vi "Umfang.vi"(9 "Breite":dbl, 10 "Länge":dbl, 11 "error in (no error)":errorcluster) -> (1 "error out":errorcluster, 2 "Umfang":dbl)   [LabVIEW 2024]
doc: "Berechnet den Umfang eines Rechteckes"
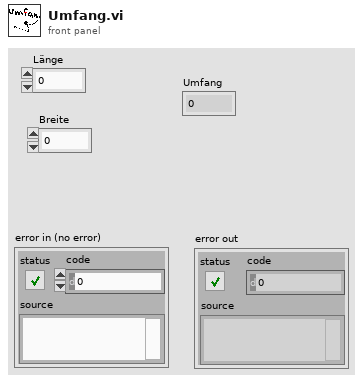
[diagram p1: front panel]
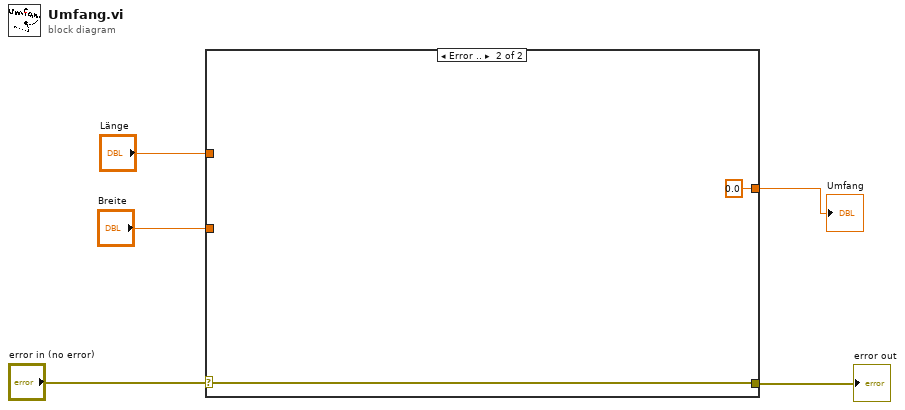
[diagram p0: block diagram]
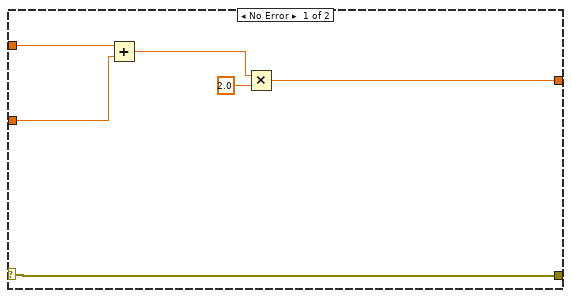
[diagram p2: hidden frame]
diagram:
  n1 = case shown="Error .." "error in (no error)" {
    selector: "error in (no error)" -> [w11 w12]
    tunnel: [w11 w12] -> w4
    tunnel: "Länge" -> [w10 _]
    tunnel: "Breite" -> [w9 _]
    tunnel: [w6 0.0] -> w1
    frame No Error {
      n2 = Add(x=w10, y=w9) -> (x+y=w8:dbl)
      n3 = Multiply(x=w8, y=2.0) -> (x*y=w6:dbl)
    }
    frame Error {
    }
  }
  "error out" <- w4
  "Umfang" <- w1
